vi "sendStartEvent.vi"(8 "error in (no error)":errorcluster) -> (0 "error out":errorcluster)   [LabVIEW 2017, in "programControl.lvlib"]
doc: "Send the start Event to all modules."
uses:
  programControl.lvlib
  StartUEFGV/TypeDefs/UEFGVcontrol.ctl
  <vilib>/event_ctls.llb/usereventprio.ctl
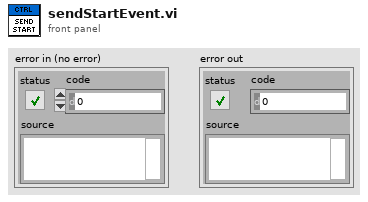
[diagram p1: front panel]
types:
  T1 = typedef "usereventprio.ctl" = enum32{"high priority", "normal priority"}
  T2 = typedef "UEFGVcontrol.ctl" = enum16{"Create", "Get", "Destroy"}
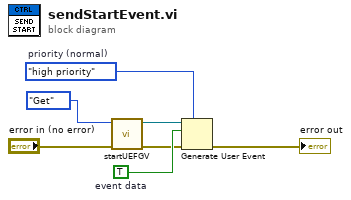
[diagram p0: block diagram]
diagram:
  w1 = usereventprio."high priority"  # priority (normal)
  w7 = TRUE  # event data
  n1 = call "startUEFGV.vi"("error in (no error)"="error in (no error)", "Enum"=UEFGVcontrol."Get") -> ("error out"=w4:errorcluster, "Start User Event"=w6:refnum<user-event>)  [unwired: 8 in]
  n2 = Generate User Event(priority (normal)=w1, user event=w6, event data cluster=w7, error in=w4) -> (error out=→"error out":errorcluster)  [unwired: 1 out]
